vi "NIDCPower_channel_ganging - configure current limit range.vi"(8 "error in (no error)":errorcluster, 9 "current limit range":dbl format="%.6p", 11 "Ganged Session In":T1) -> (0 "error out":errorcluster, 3 "Ganged Session Out":T1)   [LabVIEW 2021]
uses:
  ctl/NIDCPower_channel_ganging - ctl - ganged config.ctl
  ctl/NIDCPower_channel_ganging - ctl - channel mode.ctl
  ctl/NIDCPower_channel_ganging - ctl - ganged session.ctl
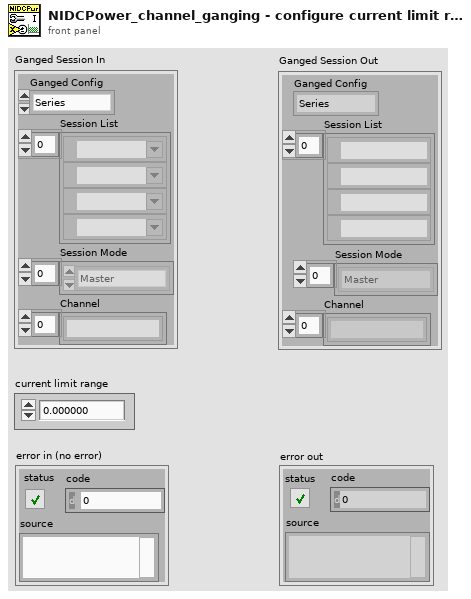
[diagram p1: front panel]
types:
  T1 = typedef "NIDCPower_channel_ganging - ctl - ganged session.ctl" = cluster{"Ganged Config":T2, "Session List":refnum<k15>[], "Session Mode":T3[], "Channel":string[]}
  T2 = typedef "NIDCPower_channel_ganging - ctl - ganged config.ctl" = enum16{"Series", "Parallel", "Manual"}
  T3 = typedef "NIDCPower_channel_ganging - ctl - channel mode.ctl" = enum16{"Master", "Slave", "Slave - Inverted"}
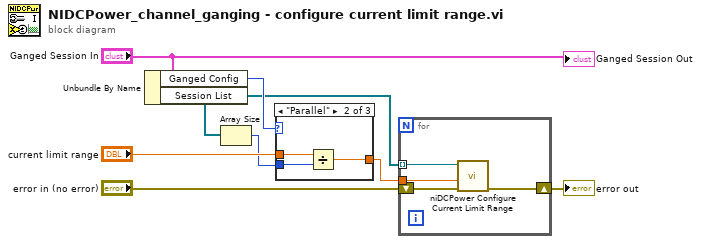
[diagram p0: block diagram]
diagram:
  n1 = Unbundle By Name("Ganged Session In") -> ("Ganged Config"=w8:T2, "Session List"=w7:refnum<k15>[])
  n2 = Array Size(array=w7) -> (size(s)=w5:i32)
  n3 = case shown="\"Parallel\"" w8 {
    tunnel: "current limit range" -> [w9 w12 w13]
    tunnel: w5 -> [_ w11 _]
    tunnel: [w9 w10 w13] -> w4
    frame "Series" {
    }
    frame "Parallel" {
      n4 = Divide(x=w12, y=w11) -> (x/y=w10:dbl)
    }
    frame "Manual" {
    }
  }
  n5 = for {
    tunnel: w7 -> [w17] mode=indexing
    tunnel: w4 -> [w16]
    shift-right: [w14] -> w2
    shift-left: "error in (no error)" -> [w15]
    n6 = call <instrlib>:"niDCPower Configure Current Limit Range.vi"("error in (no error)"=w15, "current limit range"=w16, "instrument handle"=w17) -> ("error out"=w14:errorcluster)  [unwired: 7 in, 1 out]
  }
  "error out" <- w2
  "Ganged Session Out" <- "Ganged Session In"
